vi "XYZStage-Stop all movement command.vi"(8 "Error In":errorcluster, 11 "XYZ Stage config":T1={"COM port"="COM7", "XY stage available"=FALSE}) -> (0 "Error Out":errorcluster, 1 "Move XYZ command String":string)   [LabVIEW 2013]
uses:
  Typedefs/XY Stage config cluster.ctl
  Typedefs/XYZ channel ring.ctl
  Typedefs/XYZ stage data.ctl
  Typedefs/XYZ stage states.ctl
  Globals/gl_XYZStage globals.vi
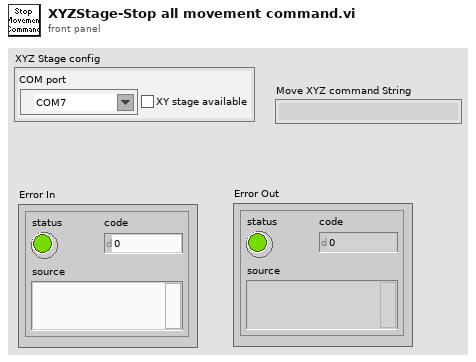
[diagram p1: front panel]
types:
  T1 = typedef "XY Stage config cluster.ctl" = cluster{"COM port":refnum<visa-resource-name>, "XY stage available":bool}
  T2 = typedef "XYZ stage data.ctl" = cluster{"Command":T3, "Channel":T4, "X":sgl, "Y":sgl, "Z":sgl, "Speed":i32, "Zero":bool, "Use acknowledgement?":bool}
  T3 = typedef "XYZ stage states.ctl" = enum16{"Dequeue", "Initialize", "Read Position", "Read Speed Setting", "Move", "Set Max Speed", "Reset Axis", "Stop all movement"}
  T4 = typedef "XYZ channel ring.ctl" = string
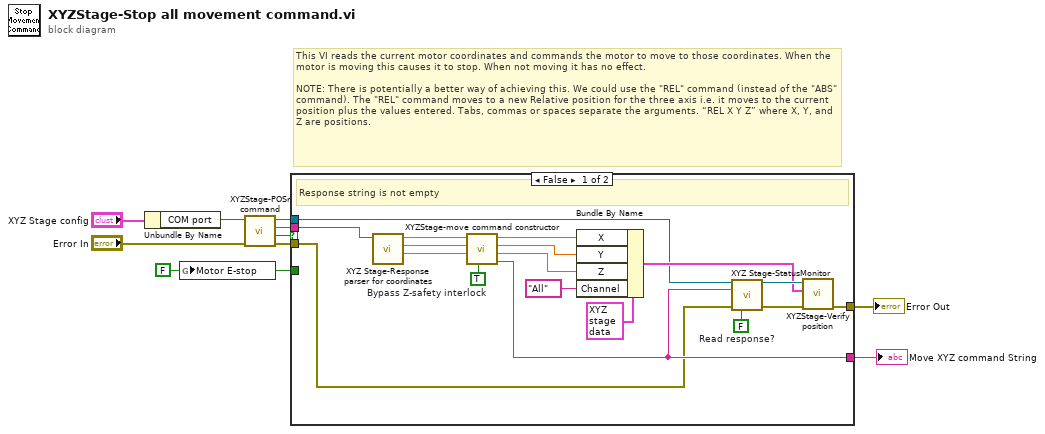
[diagram p0: block diagram]
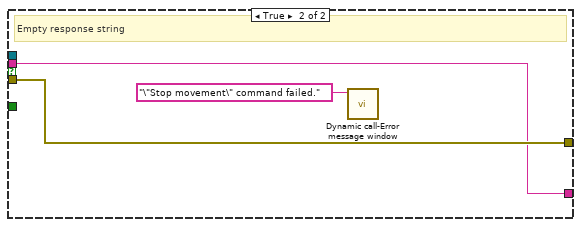
[diagram p2: hidden frame]
diagram:
  w1 = FALSE ("Motor E-stop")
  # "This VI reads the current motor coordinates and commands the motor to move to those coordinates. When the motor is moving this causes it to stop. When not moving it has no effect.\n\nNOTE: There is potentially a better way of achieving this. We could use the \"REL\" command (instead of the \"ABS\" command). The \"REL\" command moves to a new Relative position for the three axis i.e. it moves to the current position plus the values entered. Tabs, commas or spaces separate the arguments. “REL X Y Z” where X, Y, and Z are positions."
  n1 = Unbundle By Name("XYZ Stage config") -> ("COM port"=w7:refnum<visa-resource-name>)
  n2 = global write "gl_XYZStage globals.vi" "Motor E-stop"(w1) -> ()
  n3 = call "XYZStage-POSr command.vi"("Error in"="Error In", "VISA Refnum in"=w7) -> ("Error out"=w5:errorcluster, "Empty response string"=w2:bool, "read string"=w3:string, "VISA Refnum out"=w4:refnum<visa-resource-name>)  [unwired: 6 in]
  n4 = case shown="False" w2 {
    tunnel: [w27 w31] -> w9
    tunnel: [w15 w30] -> w8
    tunnel: w5 -> [w13 w31]
    tunnel: w4 -> [w12 _]
    tunnel: w3 -> [w11 w30]
    tunnel: w1 -> [_ _]
    frame False {
      w14 = TRUE  # Bypass Z-safety interlock
      w25 = FALSE  # Read response?
      # "Response string is not empty"
      n5 = call "XYZ Stage-Response parser for coordinates.vi"("Filtered response string (no CR)"=w11) -> ("Z"=w19:sgl, "Y"=w20:sgl, "X"=w21:sgl)  [unwired: 8 in]
      n6 = call "XYZStage-move command constructor.vi"("Bypass Z-safety interlock"=w14, "Z"=w19, "Y"=w20, "X"=w21) -> ("Move command"=w15:string, "Adjusted Z"=w16:sgl, "Adjusted Y"=w17:sgl, "Adjusted X"=w18:sgl)  [unwired: 4 in]
      n7 = Bundle By Name(cluster=T2 {"Command"=enum."Stop all movement", "Channel"="", "X"=0.0, "Y"=0.0, "Z"=0.0, "Speed"=0, "Zero"=TRUE, "Use acknowledgement?"=FALSE} ("XYZ Stage data"), "X"=w18, "Y"=w17, "Z"=w16, "Channel"=T4 "All") -> (w23:T2)
      n8 = call "XYZ Stage-StatusMonitor.vi"("VISA resource name"=w12, "string to write"=w15, "Error In"=w13, "Read response? (T)"=w25) -> ("VISA resource name out"=w26:refnum<visa-resource-name>, "Error Out"=w28:errorcluster)  [unwired: 7 in, 3 out]
      n9 = call "XYZStage-Verify position.vi"("error in (no error)"=w28, "XYZ Stage data"=w23, "XYZ Stage Port"=w26) -> ("error out"=w27:errorcluster)  [unwired: 8 in]
    }
    frame True {
      # "Empty response string"
      n10 = call "Dynamic call-Error message window.vi"("Error Message"="\"Stop movement\" command failed.") -> ()  [unwired: 10 in, 1 out]
    }
  }
  "Move XYZ command String" <- w8
  "Error Out" <- w9
